vi "TextFilePayload.vi"(5 "Filename":string, 9 "Content":string) -> (8 "JSON string":string)   [LabVIEW 2020, in "epl-network.lvlib"]
uses:
  epl-network.lvlib
  TextFilePayload.ctl
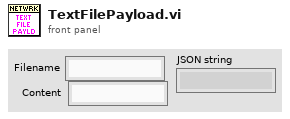
[diagram p1: front panel]
types:
  T1 = typedef "epl-network.lvlib/TextFilePayload.ctl" = cluster{"Filename":string, "Content":string}
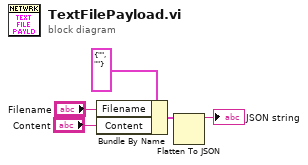
[diagram p0: block diagram]
diagram:
  n1 = Bundle By Name(cluster=T1 {"Filename"="", "Content"=""} ("TextFilePayload"), "Filename"="Filename", "Content"="Content") -> (w4:T1)
  n2 = Flatten To JSON(anything=w4) -> (JSON string=→"JSON string":string)  [unwired: 2 in, 1 out]
